vi "RecordStatus.vi"(10 "RecordStatus":u16(ring) items=["Record", "WaitingTRG", "Endless", "Recording"]) -> (1 "Color[4]":cluster{u32, u32}[](array[cluster]), 2 "String[4]":string[](array[string]), 3 "Disabled":u8)   [LabVIEW 2015]
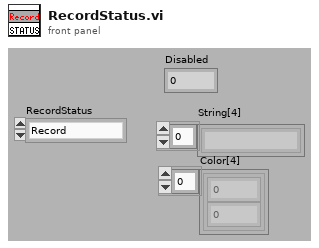
[diagram p1: front panel]
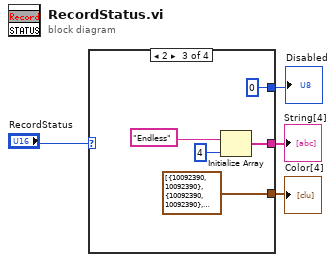
[diagram p0: block diagram]
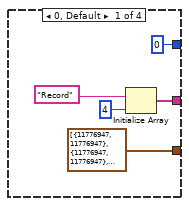
[diagram p2: hidden frame]
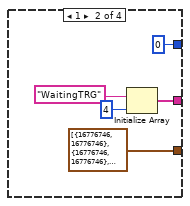
[diagram p3: hidden frame]
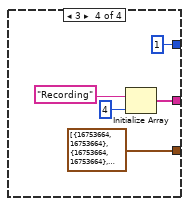
[diagram p4: hidden frame]
diagram:
  n1 = case shown="2" "RecordStatus" {
    tunnel: [w7 w12 w17 w22] -> w3
    tunnel: [cluster{u32, u32}[] [{11776947, 11776947}, {11776947, 11776947}, {8355711, 8355711}, {8355711, 8355711}] ("カラー[4]") cluster{u32, u32}[] [{16776746, 16776746}, {16776746, 16776746}, {8355711, 8355711}, {8355711, 8355711}] ("カラー[4]") cluster{u32, u32}[] [{10092390, 10092390}, {10092390, 10092390}, {8355711, 8355711}, {8355711, 8355711}] ("カラー[4]") cluster{u32, u32}[] [{16753664, 16753664}, {16753664, 16753664}, {8355711, 8355711}, {8355711, 8355711}] ("カラー[4]")] -> w2
    tunnel: [u8 0 ("Disabled") u8 0 ("Disabled") u8 0 ("Disabled") u8 1 ("Disabled")] -> w1
    frame 0, Default {
      n2 = Initialize Array("Record", 4 ("次元サイズ")) -> (w7:string[])
    }
    frame 1 {
      n3 = Initialize Array("WaitingTRG", 4 ("次元サイズ")) -> (w12:string[])
    }
    frame 2 {
      n4 = Initialize Array("Endless", 4 ("次元サイズ")) -> (w17:string[])
    }
    frame 3 {
      n5 = Initialize Array("Recording", 4 ("次元サイズ")) -> (w22:string[])
    }
  }
  "String[4]" <- w3
  "Color[4]" <- w2
  "Disabled" <- w1
